vi "rad_Retrieve Application Image From Target.vi"(5 "password":string, 7 "App Images Temp Folder":path=path "C:/dev/Architectures/Reference Designs/Application Deployment and Replication/Application Deployment Utility/trunk/source/Application Images/_temp", 8 "error in (no error)":errorcluster, 10 "Target settings":T1={"Hostname"="", "Serial number"="", "Product name"="", "Product code"=0, "System status"="", "Credential type"=enum."None/Unlocked", "User added?"=FALSE, "Primary NIC"={"MAC address"="", "IP Address Request Mode"=2, "IP address"="", "Subnet mask"="", "Gateway"="", "DNS server"=""}} {"Primary NIC"."IP Address Request Mode" items=["Static"=1, "DHCP/Link-Local"=2, "Link-Local Only"=4, "DHCP Only"=8]}, 11 "App Images Folder":path) -> (0 "error out":errorcluster, 2 "Cancelled":bool, 3 "New App Image Path":path)   [LabVIEW 2020]
uses:
  TypeDefs/rad_Retrieve Application Image States.ctl
  TypeDefs/rad_FPGA Flash Properties.ctl
  TypeDefs/rad_FPGA Properties.ctl
  TypeDefs/rad_Application Image Properties.ctl
  TypeDefs/rad_Deployment Status Data Type.ctl
  TypeDefs/rad_Deployment Progress Data Type.ctl
  TypeDefs/rad_Deployment Notifiers.ctl
  TypeDefs/rad_App Images Settings.ctl
  Targets/TypeDefs/rad_Target Information.ctl
  Targets/TypeDefs/rad_Target Network Settings.ctl
panel:
  in  "State Data":T6
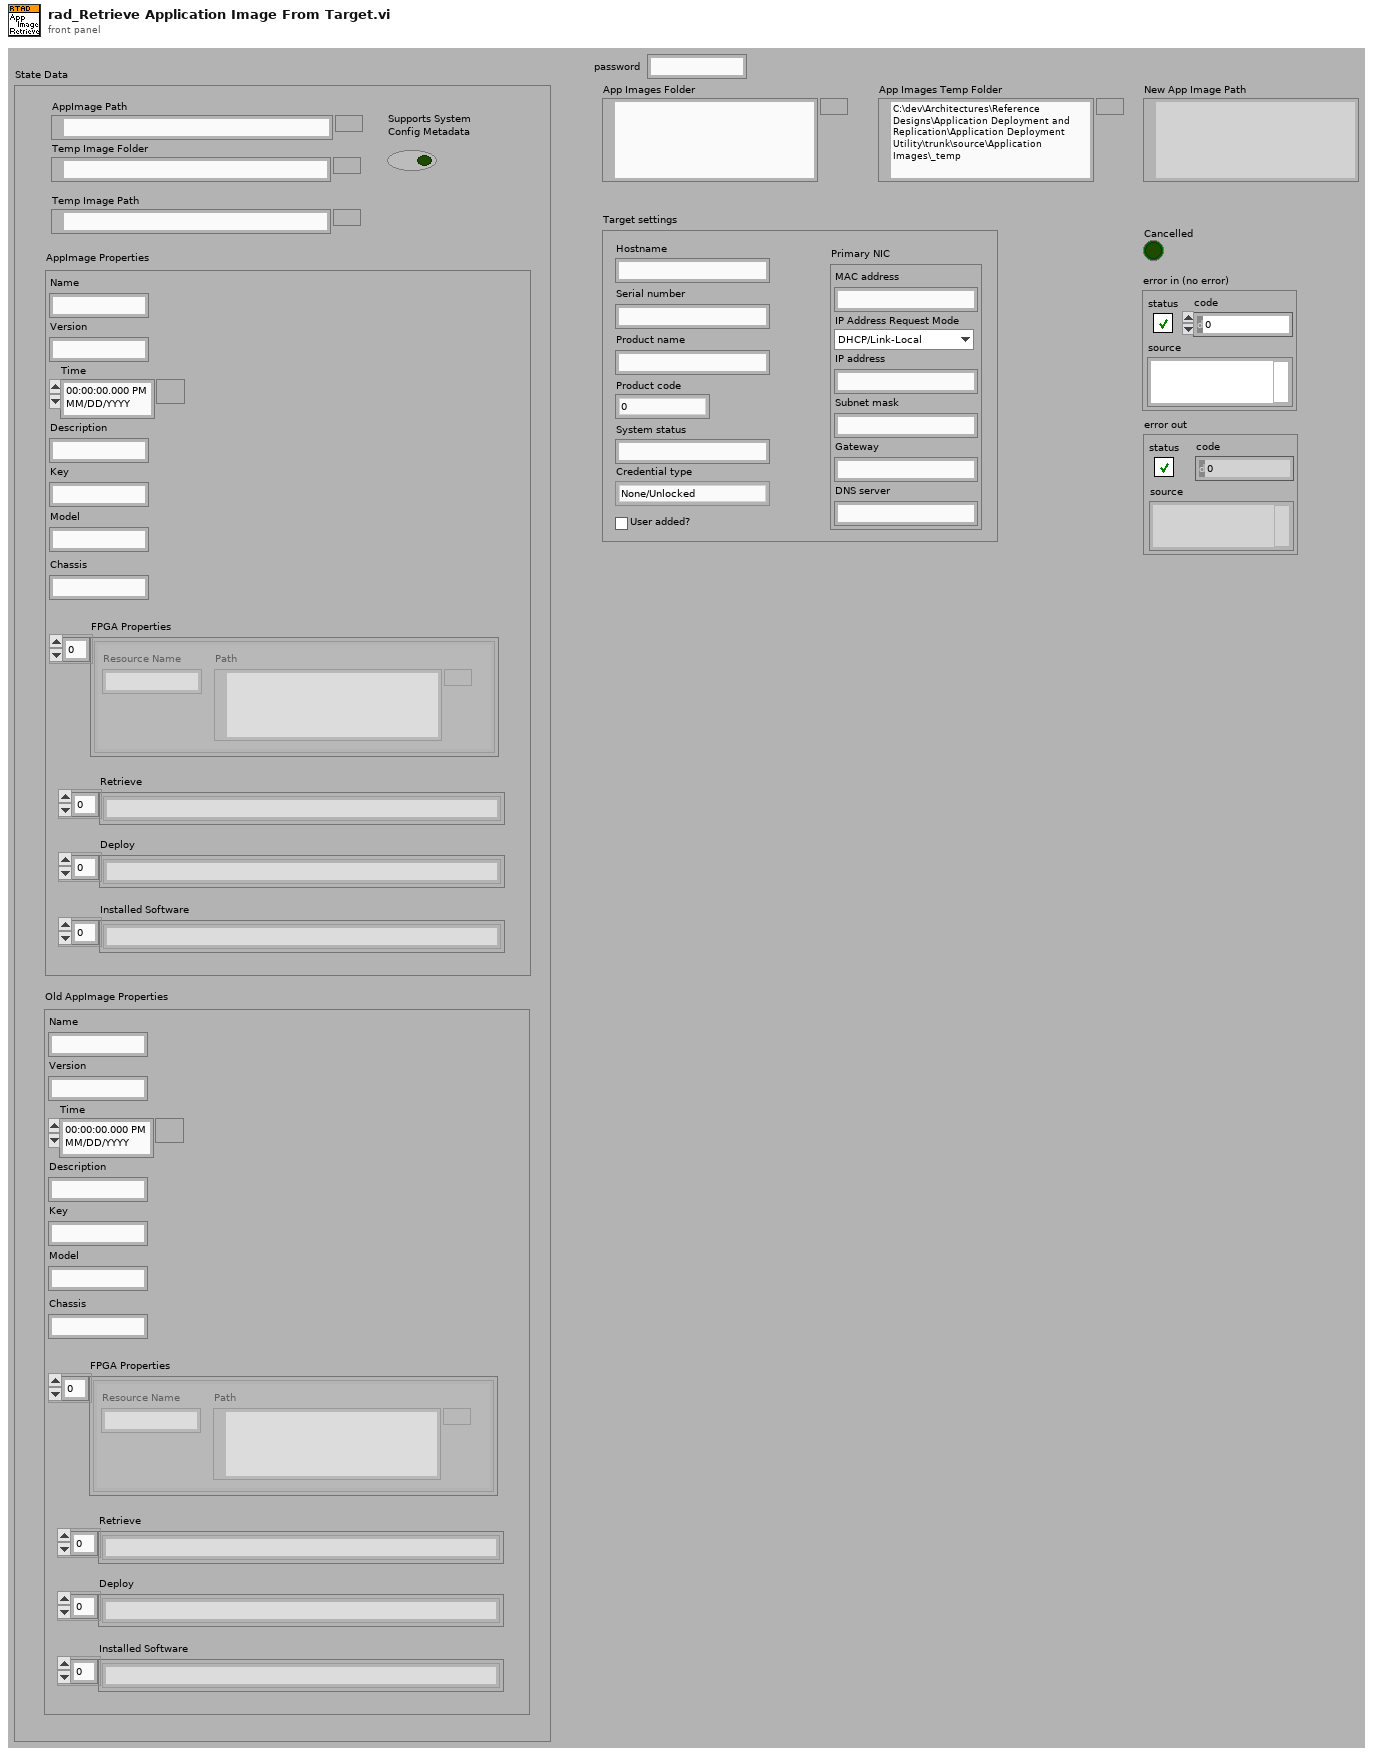
[diagram p1: front panel]
types:
  T1 = typedef "rad_Target Information.ctl" = cluster{"Hostname":string, "Serial number":string, "Product name":string, "Product code":i32, "System status":string, "Credential type":enum16{"None/Unlocked", "FTP Password", "NIAuth Credentials"}, "User added?":bool, "Primary NIC":T2}
  T2 = typedef "rad_Target Network Settings.ctl" = cluster{"MAC address":string, "IP Address Request Mode":i32, "IP address":string, "Subnet mask":string, "Gateway":string, "DNS server":string}
  T3 = typedef "rad_Application Image Properties.ctl" = cluster{"Name":string, "Version":string, "Time":timestamp, "Description":string, "Key":string, "Chassis":string, "FPGA Properties":T4, "Model":string, "Retrieve":string[], "Deploy":string[], "Installed Software":string[]}
  T4 = typedef "rad_FPGA Properties.ctl" = T5[]
  T5 = typedef "rad_FPGA Flash Properties.ctl" = cluster{"Resource Name":string, "Path":path}
  T6 = cluster{"AppImage Path":path, "Temp Image Folder":path, "AppImage Properties":T3, "App Image Info File Path":path, "New Image?":bool, "Selected Existing Image":path, "Bitfiles Modified?":bool, "Old AppImage Properties":T3, "Temp Image Path":path, "Supports System\nConfig Metadata":bool}
  T7 = typedef "rad_Retrieve Application Image States.ctl" = enum16{"Verify App Image Directory", "Get Target's Image Info", "Select Image Prop. Source", "Find Existing Disk Image", "Get Disk Image Properties", "Create New Image", "Set Image Properties", "Get Image Save Location", "GetInstalledSoftware", "Create App Image Info File", "Deploy New Files to Target", "Retrieve Application Image", "PackageImage", "Cleanup", "Exit"}
  T8 = typedef "rad_App Images Settings.ctl" = cluster{"App Images Folder":path, "App Images Temp Folder":path, "CurrentVersion":string}
  T9 = enum16{"None/Unlocked", "FTP Password", "NIAuth Credentials"}
  T10 = typedef "rad_Deployment Notifiers.ctl" = cluster{"Status":refnum<notifier>, "Progress":refnum<notifier>}
  T11 = typedef "rad_Deployment Progress Data Type.ctl" = i8
  T12 = typedef "rad_Deployment Status Data Type.ctl" = string
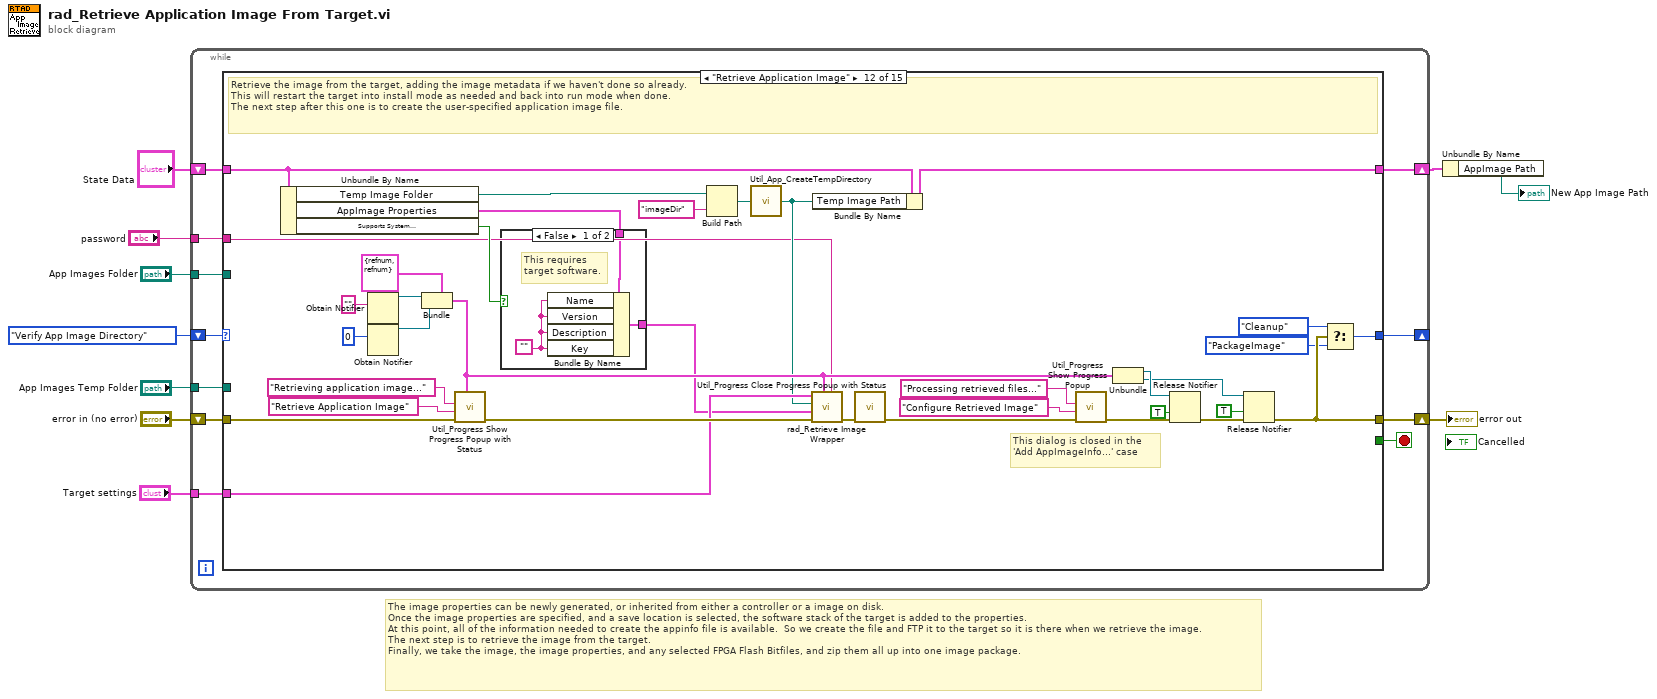
[diagram p0: block diagram]
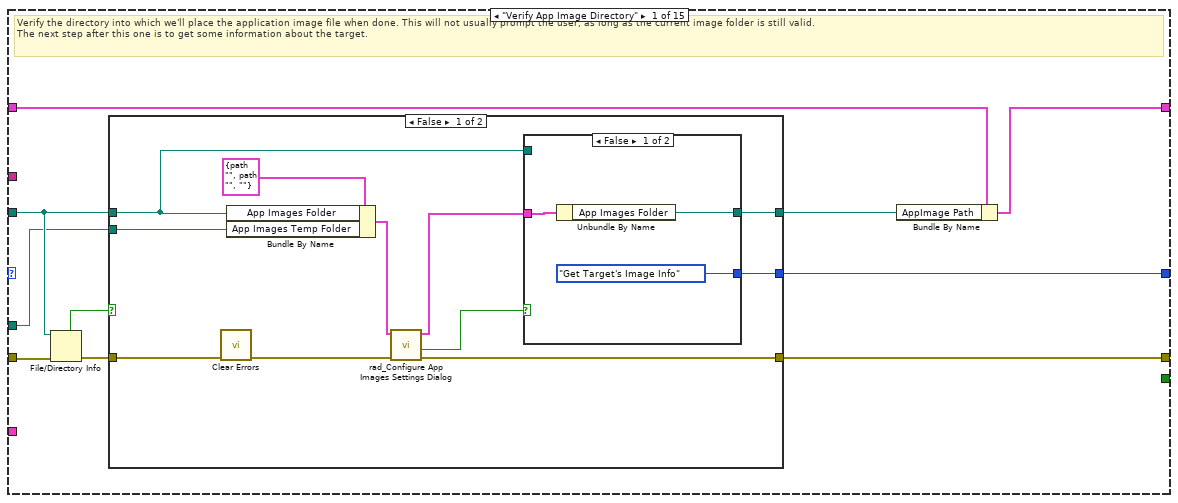
[diagram p2: hidden frame]
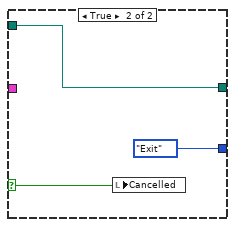
[diagram p3: hidden frame]
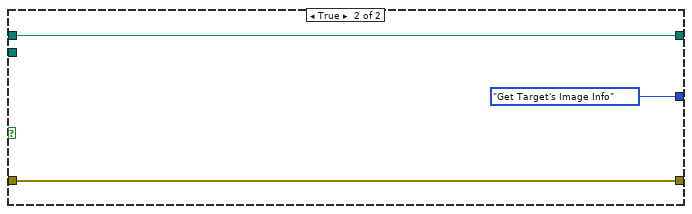
[diagram p4: hidden frame]
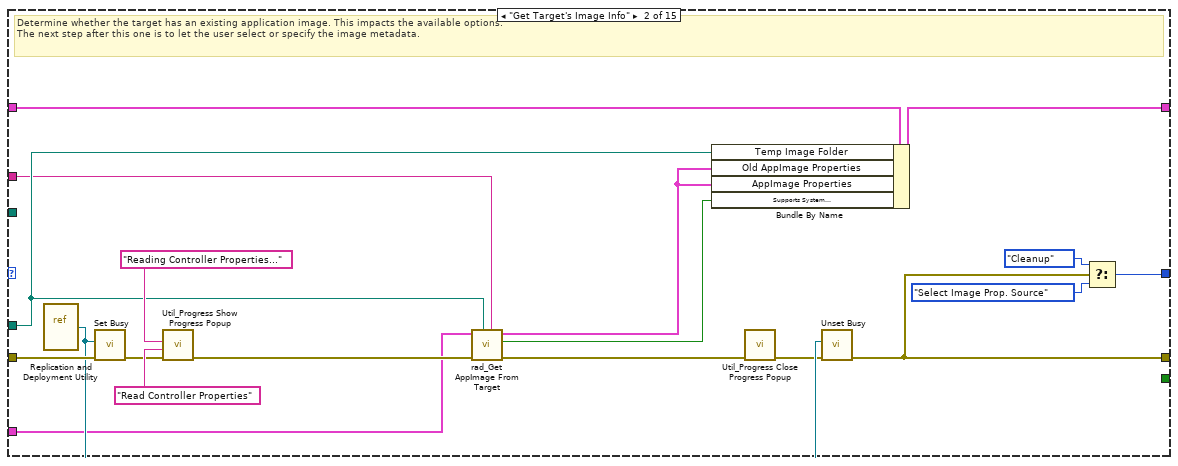
[diagram p5: hidden frame]
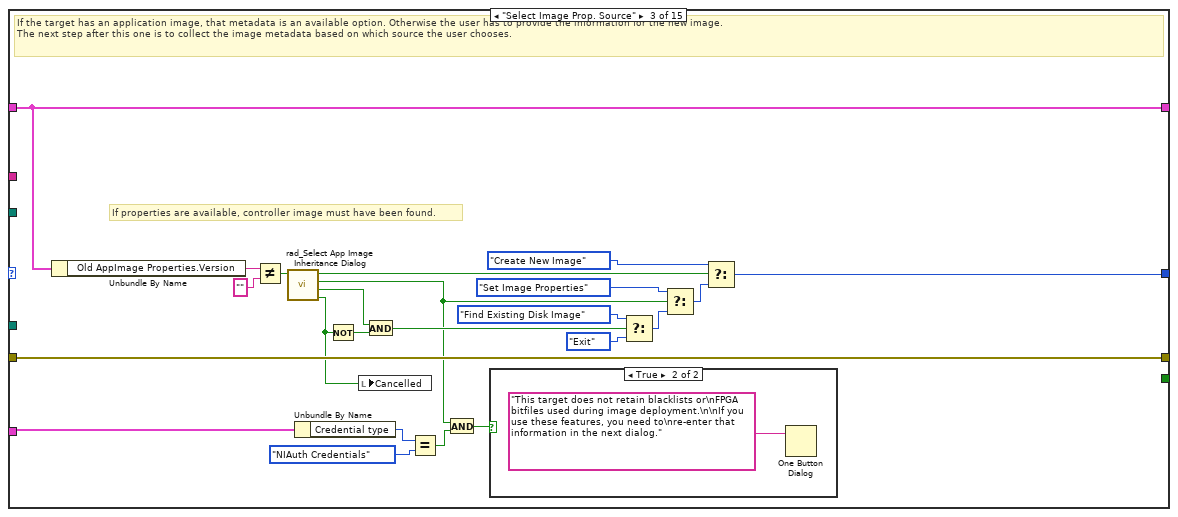
[diagram p6: hidden frame]
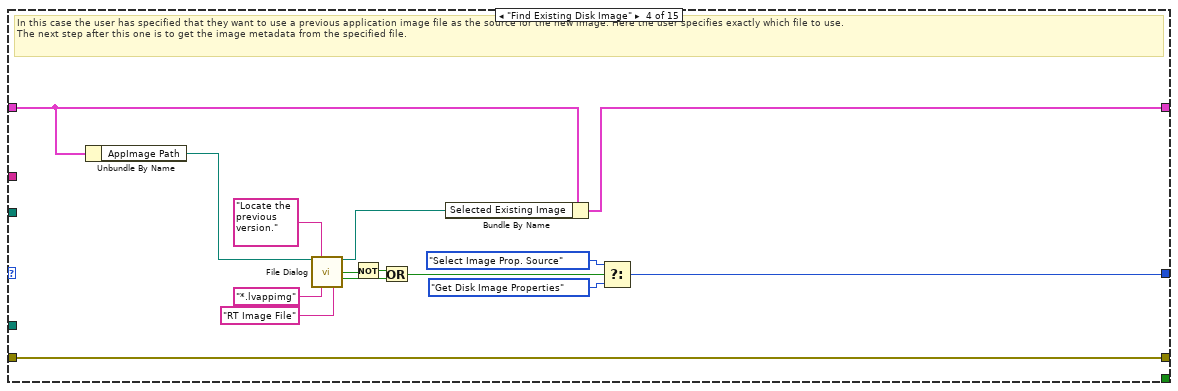
[diagram p8: hidden frame]
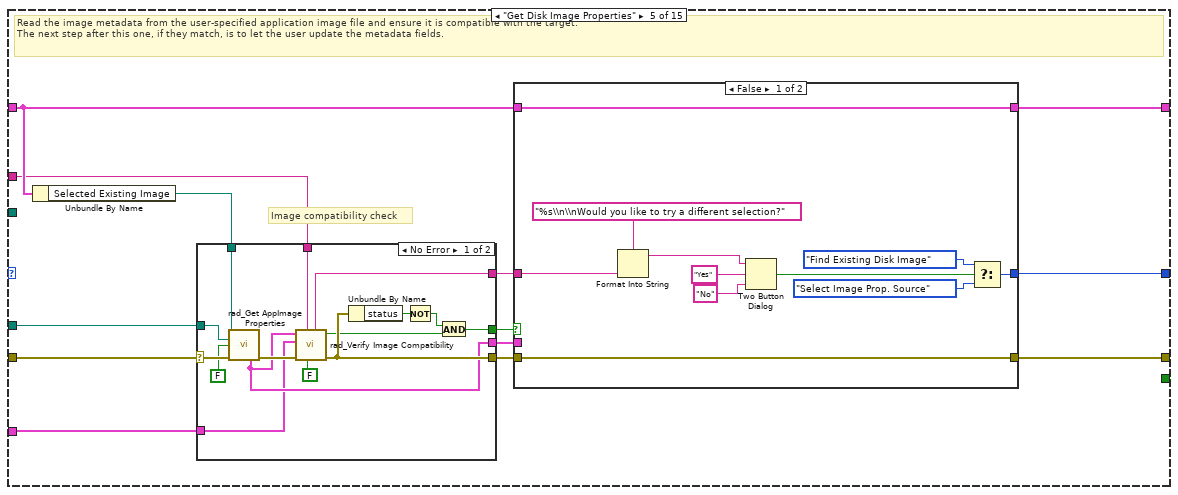
[diagram p9: hidden frame]
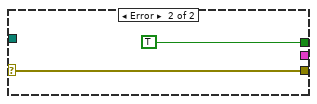
[diagram p10: hidden frame]
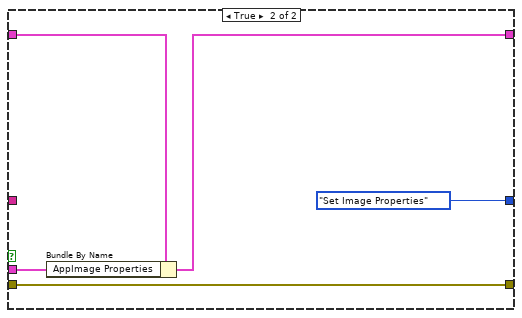
[diagram p11: hidden frame]
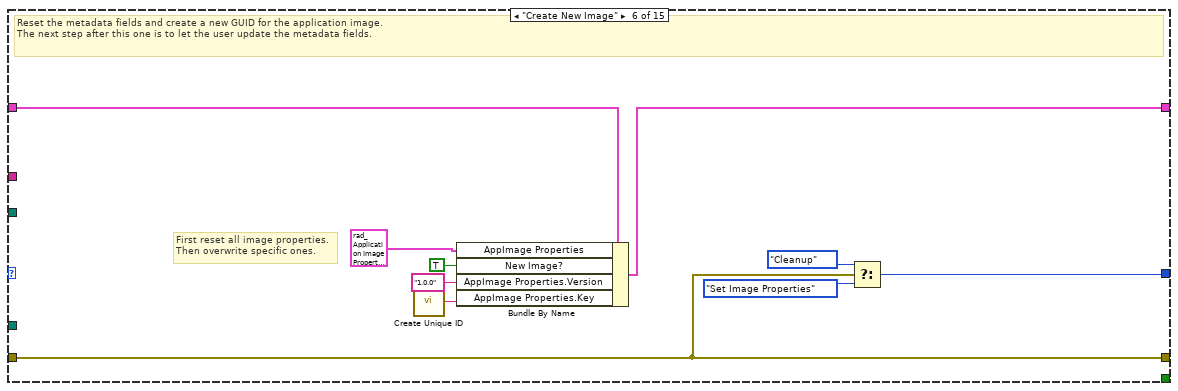
[diagram p12: hidden frame]
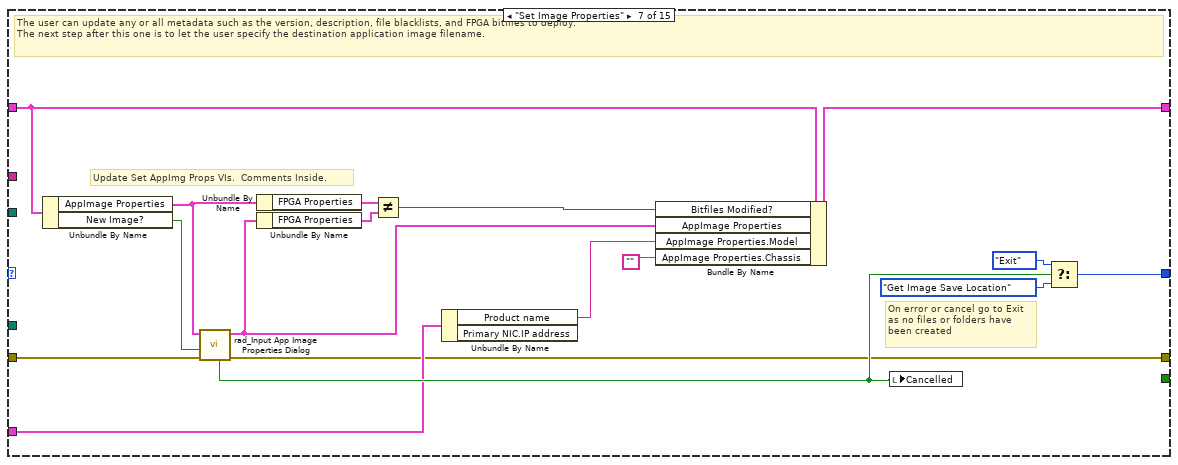
[diagram p13: hidden frame]
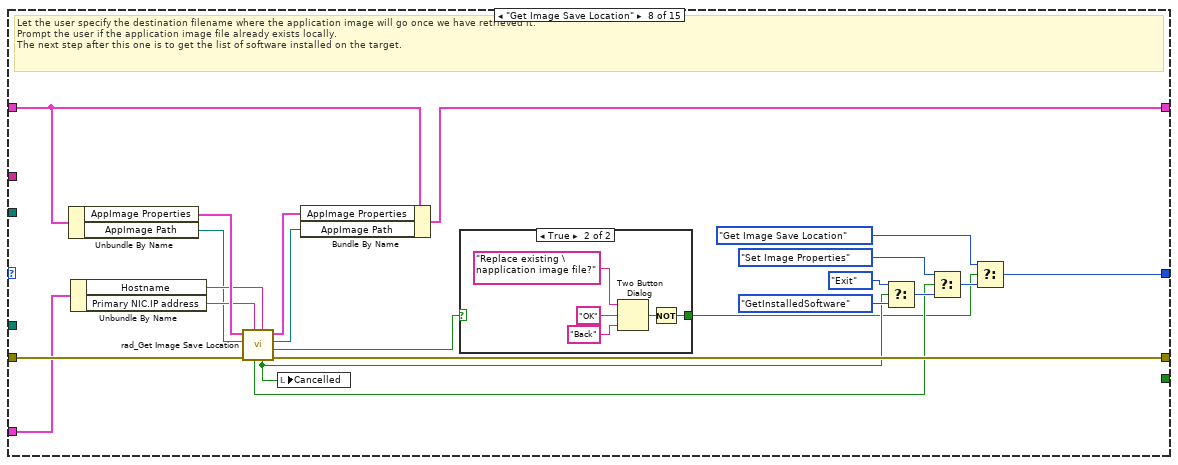
[diagram p14: hidden frame]
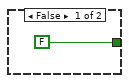
[diagram p15: hidden frame]
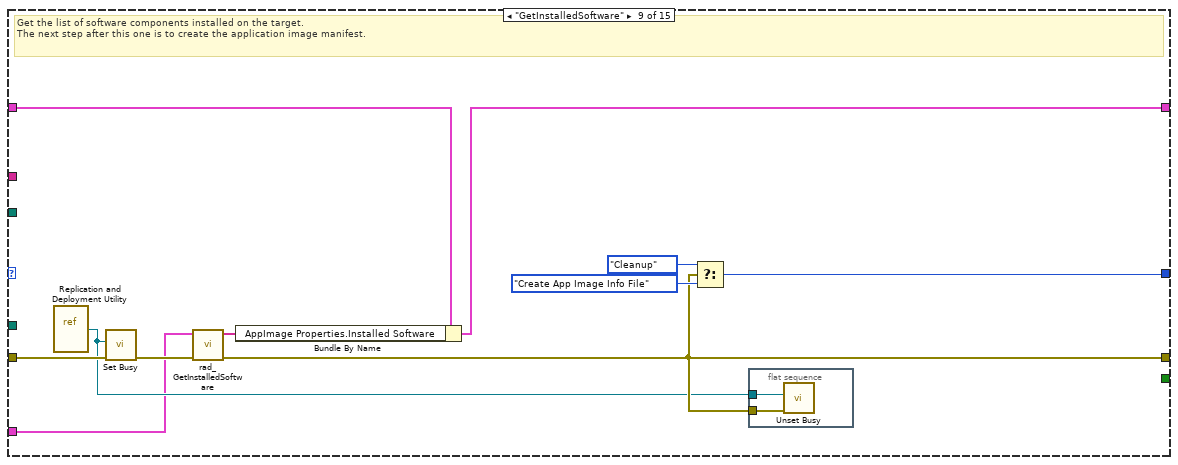
[diagram p16: hidden frame]
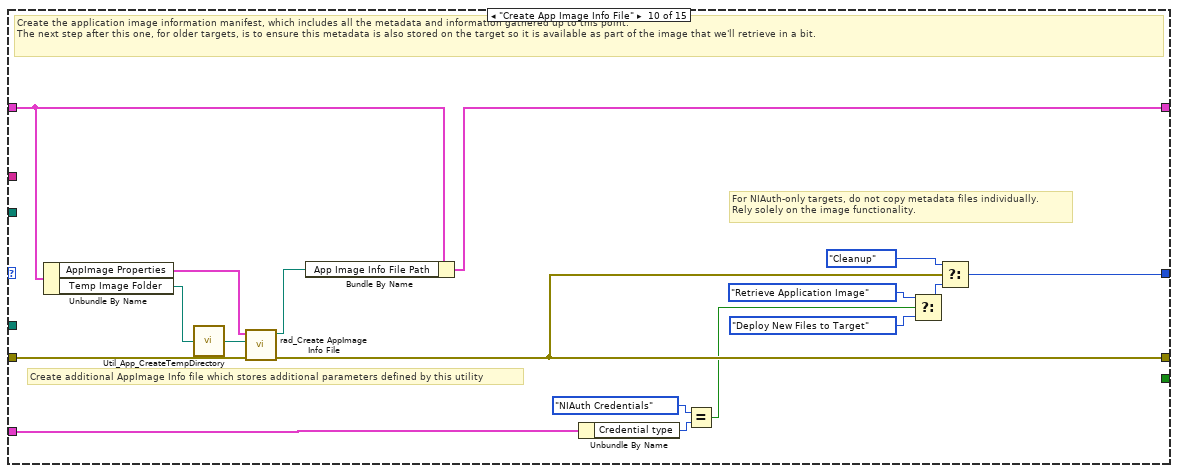
[diagram p17: hidden frame]
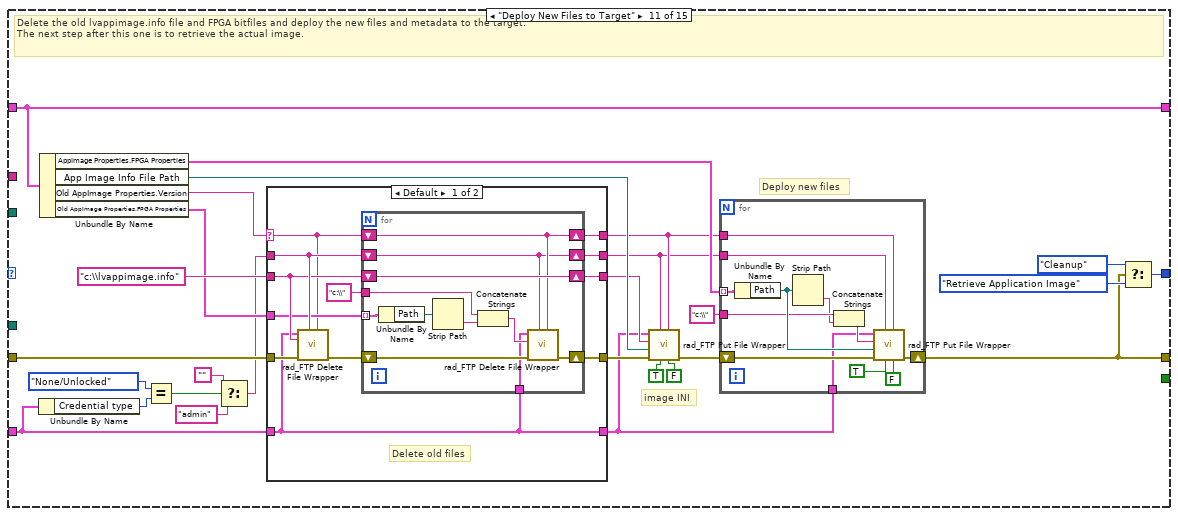
[diagram p18: hidden frame]
diagram:
  # "The image properties can be newly generated, or inherited from either a controller or a image on disk.\nOnce the image properties are specified, and a save location is selected, the software stack of the target is added to the properties.\nAt this point, all of the information needed to create the appinfo file is available.  So we create the file and FTP it to the target so it is there when we retrieve the image.\nThe next step is to retrieve the image from the target.\nFinally, we take the image, the image properties, and any selected FPGA Flash Bitfiles, and zip them all up into one image package."
  n1 = while {
    shift-right: [w20] -> _
    shift-left: rad_Retrieve_Application_Image_States."Verify App Image Directory" ("Retrieve App Images States") -> [w21]
    shift-right: [w17] -> w6
    shift-left: "State Data" -> [w18]
    shift-right: [w15] -> w7
    shift-left: "error in (no error)" -> [w16]
    tunnel: "App Images Folder" -> [w14]
    tunnel: "App Images Temp Folder" -> [w13]
    tunnel: "Target settings" -> [w12]
    tunnel: "password" -> [w11]
    stop <- w19 stop-if-true
    n2 = case shown="\"Retrieve Application Image\"" w21 {
      tunnel: [w25 w69 w81 w108 w121 w162 w182 w188 w217 w240 w252 w341 rad_Retrieve_Application_Image_States."Cleanup" ("Retrieve App Images States") rad_Retrieve_Application_Image_States."Exit" ("Retrieve App Images States") _] -> w20
      tunnel: [_ _ _ _ _ _ _ _ _ _ _ _ _ _ TRUE] -> w19
      tunnel: w18 -> [w24 w64 w93 w96 w118 w158 w177 w202 w220 w235 w267 w339 w351 w361 w375]
      tunnel: [w23 w68 w93 w107 w114 w165 w178 w201 w219 w237 w267 w340 w351 w361 w375] -> w17
      tunnel: w16 -> [w31 w63 w82 w109 w120 w156 w181 w204 w214 w233 w257 w334 w353 w355 w378]
      tunnel: [w28 w61 w82 w109 w116 w156 w167 w197 w215 w238 w251 w322 w352 w357 w378] -> w15
      tunnel: w14 -> [w27 _ _ _ _ _ _ _ _ _ _ _ _ _ _]
      tunnel: w13 -> [w26 w54 _ _ w115 _ _ _ _ _ _ _ _ _ _]
      tunnel: w12 -> [_ w55 w76 _ w111 _ w168 w186 w211 w227 w248 w315 _ _ _]
      tunnel: w11 -> [_ w52 _ _ w110 _ _ _ _ _ _ w308 _ _ _]
      frame "Verify App Image Directory" {
        # "Verify the directory into which we'll place the application image file when done. This will not usually prompt the user, as long as the current image folder is still valid.\nThe next step after this one is to get some information about the target."
        n3 = File/Directory Info(path=w27, error in=w31) -> (directory=w30:bool, error out=w29:errorcluster)  [unwired: 5 out]
        n4 = case shown="False" w30 {
          tunnel: w29 -> [w42 w51]
          tunnel: [w40 w51] -> w28
          tunnel: w27 -> [w32 w49]
          tunnel: w26 -> [w41 _]
          tunnel: [w37 rad_Retrieve_Application_Image_States."Get Target's Image Info" ("Retrieve App Images States")] -> w25
          tunnel: [w33 w49] -> w22
          frame False {
            n5 = call <vilib>:"Clear Errors.vi"("error in (no error)"=w42) -> ("error out"=w34:errorcluster)  [unwired: 5 in, 1 out]
            n6 = Bundle By Name(cluster=T8 {"App Images Folder"=path "", "App Images Temp Folder"=path "", "CurrentVersion"=""} ("App Images Settings"), "App Images Folder"=w32, "App Images Temp Folder"=w41) -> (w35:T8)
            n7 = call "rad_Configure App Images Settings Dialog.vi"("error in (no error)"=w34, "App Images Settings"=w35) -> ("error out"=w40:errorcluster, "Cancelled"=w39:bool, "App Images Settings"=w38:T8)  [unwired: 7 out]
            n8 = case shown="False" w39 {
              selector: w39 -> [_ w46]
              tunnel: w38 -> [w44 _]
              tunnel: [rad_Retrieve_Application_Image_States."Get Target's Image Info" ("Retrieve App Images States") rad_Retrieve_Application_Image_States."Exit" ("Retrieve App Images States")] -> w37
              tunnel: [w43 w47] -> w33
              tunnel: w32 -> [_ w47]
              frame False {
                n9 = Unbundle By Name(w44) -> ("App Images Folder"=w43:path)
              }
              frame True {
                n10 = local write "Cancelled"(w46) -> ()
              }
            }
          }
          frame True {
          }
        }
        n11 = Bundle By Name(cluster=w24, "AppImage Path"=w22) -> (w23:T6)
      }
      frame "Get Target's Image Info" {
        # "Determine whether the target has an existing application image. This impacts the available options.\nThe next step after this one is to let the user select or specify the image metadata."
        n12 = vi-ref "Replication and Deployment Utility.vi"() -> (w60:refnum<vi>)
        n13 = call <vilib>:"Set Busy.vi"("error in (no error)"=w63, "VI reference (current VI)"=w60) -> ("error out"=w62:errorcluster)  [unwired: 8 in, 1 out]
        n14 = call "Util_Progress Show Progress Popup.vi"("error in (no error)"=w62, "Title"="Read Controller Properties", "Message"="Reading Controller Properties...") -> ("error out"=w58:errorcluster)  [unwired: 8 in]
        n15 = call "rad_Get AppImage From Target.vi"("password"=w52, "Temp Folder"=w54, "error in (no error)"=w58, "Target settings"=w55) -> ("error out"=w57:errorcluster, "Supports System\nConfig Metadata"=w53:bool, "AppImage Properties"=w56:T3)  [unwired: 5 in]
        n16 = Bundle By Name(cluster=w64, "Temp Image Folder"=w54, "Old AppImage Properties"=w56, "AppImage Properties"=w56, "Supports System\nConfig Metadata"=w53) -> (w68:T6)
        n17 = call "Util_Progress Close Progress Popup.vi"("error in (no error)"=w57) -> ("error out"=w59:errorcluster)  [unwired: 10 in]
        n18 = call <vilib>:"Unset Busy.vi"("error in (no error)"=w59, "VI reference (current VI)"=w60) -> ("error out"=w61:errorcluster)  [unwired: 9 in]
        n19 = Select(t=rad_Retrieve_Application_Image_States."Cleanup", s=w61, f=rad_Retrieve_Application_Image_States."Select Image Prop. Source" ("Retrieve App Images States")) -> (s? t:f=w69:T7)
      }
      frame "Select Image Prop. Source" {
        # "If properties are available, controller image must have been found."
        # "If the target has an application image, that metadata is an available option. Otherwise the user has to provide the information for the new image.\nThe next step after this one is to collect the image metadata based on which source the user chooses."
        n20 = Unbundle By Name(w93) -> ("Old AppImage Properties.Version"=w92:string)
        n21 = Not Equal?(x=w92, y="") -> (x != y?=w90:bool)
        n22 = call "rad_Select App Image Inheritance Dialog.vi"("Controller Image Available?"=w90) -> ("Cancel"=w77:bool, "Disc Image"=w80:bool, "Controller Image"=w72:bool, "New Image"=w89:bool)  [unwired: 7 in]
        n23 = Unbundle By Name(w76) -> ("Credential type"=w75:T9)
        n24 = Not(x=w77) -> (.not. x?=w79:bool)
        n25 = local write "Cancelled"(w77) -> ()
        n26 = And(x=w80, y=w79) -> (x .and. y?=w78:bool)
        n27 = Equal?(x=w75, y=T9."NIAuth Credentials" ("Credential type")) -> (x = y?=w73:bool)
        n28 = And(x=w72, y=w73) -> (x .and. y?=w71:bool)
        n29 = case shown="True" w71 {
          frame False {
          }
          frame True {
            n30 = One Button Dialog(message="This target does not retain blacklists or\nFPGA bitfiles used during image deployment.\n\nIf you use these features, you need to\nre-enter that information in the next dialog.") -> ()  [unwired: 1 in, 1 out]
          }
        }
        n31 = Select(t=rad_Retrieve_Application_Image_States."Find Existing Disk Image" ("Retrieve App Images States"), s=w78, f=rad_Retrieve_Application_Image_States."Exit" ("Retrieve App Images States")) -> (s? t:f=w84:T7)
        n32 = Select(t=rad_Retrieve_Application_Image_States."Set Image Properties" ("Retrieve App Images States"), s=w72, f=w84) -> (s? t:f=w86:T7)
        n33 = Select(t=rad_Retrieve_Application_Image_States."Create New Image" ("Retrieve App Images States"), s=w89, f=w86) -> (s? t:f=w81:T7)
      }
      frame "Find Existing Disk Image" {
        # "In this case the user has specified that they want to use a previous application image file as the source for the new image. Here the user specifies exactly which file to use.\nThe next step after this one is to get the image metadata from the specified file."
        n34 = Unbundle By Name(w96) -> ("AppImage Path"=w95:path)
        n35 = call "File Dialog"("start path"=w95, "prompt"="Locate the previous version.", "pattern (all files)"="*.lvappimg", "pattern label"="RT Image File") -> ("selected path"=w97:path, "exists"=w104:bool, "cancelled"=w102:bool)  [unwired: 8 in, 1 out]
        n36 = Not(x=w104) -> (.not. x?=w103:bool)
        n37 = Or(x=w103, y=w102) -> (x .or. y?=w100:bool)
        n38 = Bundle By Name(cluster=w96, "Selected Existing Image"=w97) -> (w107:T6)
        n39 = Select(t=rad_Retrieve_Application_Image_States."Select Image Prop. Source" ("f"), s=w100, f=rad_Retrieve_Application_Image_States."Get Disk Image Properties") -> (s? t:f=w108:T7)
      }
      frame "Get Disk Image Properties" {
        # "Image compatibility check"
        # "Read the image metadata from the user-specified application image file and ensure it is compatible with the target.\nThe next step after this one, if they match, is to let the user update the metadata fields."
        n40 = Unbundle By Name(w118) -> ("Selected Existing Image"=w122:path)
        n41 = case shown="No Error" w120 {
          selector: w120 -> [w129 w139]
          tunnel: w115 -> [w130 _]
          tunnel: w122 -> [w131 _]
          tunnel: [w137 w139] -> w117
          tunnel: [w135 TRUE] -> w119
          tunnel: [w126 _] -> w113
          tunnel: w111 -> [w125 _]
          tunnel: [w124 _] -> w112
          tunnel: w110 -> [w123 _]
          frame No Error {
            n42 = call "rad_Get AppImage Properties.vi"("AppImage Path"=w131, "App Image Temp Folder"=w130, "Show FP"=FALSE, "error in (no error)"=w129) -> ("AppImage Properties"=w126:T3, "error out"=w128:errorcluster)  [unwired: 5 in, 5 out]
            n43 = call "rad_Verify Image Compatibility.vi"("Require Identical Chassis?"=FALSE, "Password"=w123, "error in (no error)"=w128, "Target address"=w125, "AppImage Properties"=w126) -> ("error out"=w137:errorcluster, "Compatible?"=w134:bool, "Status message"=w124:string)  [unwired: 4 in]
            n44 = Unbundle By Name(w137) -> ("status"=w136:bool)
            n45 = Not(x=w136) -> (.not. x?=w133:bool)
            n46 = And(x=w133, y=w134) -> (x .and. y?=w135:bool)
          }
          frame Error {
          }
        }
        n47 = case shown="False" w119 {
          tunnel: [w145 rad_Retrieve_Application_Image_States."Set Image Properties" ("Retrieve App Images States")] -> w121
          tunnel: w118 -> [w143 w155]
          tunnel: w117 -> [w144 w151]
          tunnel: [w144 w151] -> w116
          tunnel: [w143 w153] -> w114
          tunnel: w113 -> [_ w152]
          tunnel: w112 -> [w141 _]
          frame False {
            n48 = Format Into String(format string="%s\\n\\nWould you like to try a different selection?" ("message"), w141) -> (resulting string=w140:string)  [unwired: 2 in, 1 out]
            n49 = Two Button Dialog(message=w140, 1:"No" ("F button name (\"Cancel\")"), 2:"Yes" ("T button name (\"OK\")")) -> (T button?=w147:bool)
            n50 = Select(t=rad_Retrieve_Application_Image_States."Find Existing Disk Image" ("Retrieve App Images States"), s=w147, f=rad_Retrieve_Application_Image_States."Select Image Prop. Source" ("Retrieve App Images States")) -> (s? t:f=w145:T7)
          }
          frame True {
            n51 = Bundle By Name(cluster=w155, "AppImage Properties"=w152) -> (w153:T6)
          }
        }
      }
      frame "Create New Image" {
        # "First reset all image properties.\nThen overwrite specific ones."
        # "Reset the metadata fields and create a new GUID for the application image.\nThe next step after this one is to let the user update the metadata fields."
        n52 = call "Create Unique ID.vi"() -> ("ID String"=w161:string)  [unwired: 1 in]
        n53 = Bundle By Name(cluster=w158, "AppImage Properties"=T3 {"Name"="", "Version"="", "Time"=timestamp(0 s since 1904-01-01), "Description"="", "Key"="", "Chassis"="", "FPGA Properties"=[], "Model"="", "Retrieve"=[], "Deploy"=[], "Installed Software"=[]}, "New Image?"=TRUE, "AppImage Properties.Version"="1.0.0", "AppImage Properties.Key"=w161) -> (w165:T6)
        n54 = Select(t=rad_Retrieve_Application_Image_States."Cleanup", s=w156, f=rad_Retrieve_Application_Image_States."Set Image Properties" ("Retrieve App Images States")) -> (s? t:f=w162:T7)
      }
      frame "Set Image Properties" {
        # "Update Set AppImg Props VIs.  Comments Inside."
        # "On error or cancel go to Exit\nas no files or folders have\nbeen created"
        # "The user can update any or all metadata such as the version, description, file blacklists, and FPGA bitfiles to deploy.\nThe next step after this one is to let the user specify the destination application image filename."
        n55 = Unbundle By Name(w177) -> ("AppImage Properties"=w172:T3, "New Image?"=w173:bool)
        n56 = call "rad_Input App Image Properties Dialog.vi"("error in (no error)"=w181, "New Image?"=w173, "AppImage Properties"=w172) -> ("error out"=w167:errorcluster, "AppImage Properties"=w170:T3, "Cancelled"=w171:bool)  [unwired: 4 in, 2 out]
        n57 = Unbundle By Name(w172) -> ("FPGA Properties"=w176:T4)
        n58 = Unbundle By Name(w170) -> ("FPGA Properties"=w175:T4)
        n59 = Not Equal?(x=w176, y=w175) -> (x != y?=w174:bool)
        n60 = Unbundle By Name(w168) -> ("Product name"=w169:string)  [unwired: 1 out]
        n61 = Bundle By Name(cluster=w177, "Bitfiles Modified?"=w174, "AppImage Properties"=w170, "AppImage Properties.Model"=w169, "AppImage Properties.Chassis"="") -> (w178:T6)
        n62 = local write "Cancelled"(w171) -> ()
        n63 = Select(t=rad_Retrieve_Application_Image_States."Exit" ("Retrieve App Images States"), s=w171, f=rad_Retrieve_Application_Image_States."Get Image Save Location" ("Retrieve App Images States")) -> (s? t:f=w182:T7)
      }
      frame "Get Image Save Location" {
        # "Let the user specify the destination filename where the application image will go once we have retrieved it.\nPrompt the user if the application image file already exists locally.\nThe next step after this one is to get the list of software installed on the target."
        n64 = Unbundle By Name(w202) -> ("AppImage Properties"=w203:T3, "AppImage Path"=w183:path)
        n65 = Unbundle By Name(w186) -> ("Hostname"=w185:string, "Primary NIC.IP address"=w184:string)
        n66 = call "rad_Get Image Save Location.vi"("Host Name"=w185, "IP Address"=w184, "error in (no error)"=w204, "Starting Path"=w183, "AppImage Properties"=w203) -> ("error out"=w197:errorcluster, "exists"=w198:bool, "Application Image Path"=w192:path, "AppImage Properties"=w200:T3, "Cancelled"=w191:bool, "Back"=w194:bool)  [unwired: 1 in]
        n67 = local write "Cancelled"(w191) -> ()
        n68 = Bundle By Name(cluster=w202, "AppImage Properties"=w200, "AppImage Path"=w192) -> (w201:T6)
        n69 = case shown="True" w198 {
          tunnel: [FALSE ("T button?") w206] -> w189
          frame False {
          }
          frame True {
            n70 = Two Button Dialog(message="Replace existing \napplication image file?", 1:"Back" ("F button name (\"Cancel\")"), 2:"OK" ("T button name (\"OK\")")) -> (T button?=w209:bool)
            n71 = Not(x=w209) -> (.not. x?=w206:bool)
          }
        }
        n72 = Select(t=rad_Retrieve_Application_Image_States."Exit" ("Retrieve App Images States"), s=w191, f=rad_Retrieve_Application_Image_States."GetInstalledSoftware" ("Retrieve App Images States")) -> (s? t:f=w195:T7)
        n73 = Select(t=rad_Retrieve_Application_Image_States."Set Image Properties", s=w194, f=w195) -> (s? t:f=w190:T7)
        n74 = Select(t=rad_Retrieve_Application_Image_States."Get Image Save Location", s=w189, f=w190) -> (s? t:f=w188:T7)
      }
      frame "GetInstalledSoftware" {
        # "Get the list of software components installed on the target.\nThe next step after this one is to create the application image manifest."
        n75 = vi-ref "Replication and Deployment Utility.vi"() -> (w212:refnum<vi>)
        n76 = call <vilib>:"Set Busy.vi"("error in (no error)"=w214, "VI reference (current VI)"=w212) -> ("error out"=w213:errorcluster)  [unwired: 8 in, 1 out]
        n77 = call "rad_GetInstalledSoftware.vi"("error in (no error)"=w213, "Target settings"=w211) -> ("error out"=w215:errorcluster, "installedSoftware"=w221:string[])  [unwired: 8 in]
        n78 = Bundle By Name(cluster=w220, "AppImage Properties.Installed Software"=w221) -> (w219:T6)
        n79 = Select(t=rad_Retrieve_Application_Image_States."Cleanup", s=w215, f=rad_Retrieve_Application_Image_States."Create App Image Info File" ("Retrieve App Images States")) -> (s? t:f=w217:T7)
        n80 = flat-sequence {
          tunnel: w215 -> [w223]
          tunnel: w212 -> [w222]
          frame #0 {
            n81 = call <vilib>:"Unset Busy.vi"("error in (no error)"=w223, "VI reference (current VI)"=w222) -> ()  [unwired: 9 in, 1 out]
          }
        }
      }
      frame "Create App Image Info File" {
        # "For NIAuth-only targets, do not copy metadata files individually.\nRely solely on the image functionality."
        # "Create additional AppImage Info file which stores additional parameters defined by this utility"
        # "Create the application image information manifest, which includes all the metadata and information gathered up to this point.\nThe next step after this one, for older targets, is to ensure this metadata is also stored on the target so it is available as part of the image that we'll retrieve in a bit."
        n82 = Unbundle By Name(w235) -> ("AppImage Properties"=w234:T3, "Temp Image Folder"=w224:path)
        n83 = call "Util_App_CreateTempDirectory.vi"("TempFolderPath"=w224) -> ("TempFolderPath_out"=w232:path)
        n84 = call "rad_Create AppImage Info File.vi"("error in (no error)"=w233, "Temp Image Folder"=w232, "AppImage Properties"=w234) -> ("error out"=w238:errorcluster, "App Image Info file path"=w236:path)  [unwired: 7 in]
        n85 = Bundle By Name(cluster=w235, "App Image Info File Path"=w236) -> (w237:T6)
        n86 = Unbundle By Name(w227) -> ("Credential type"=w229:T9)
        n87 = Equal?(x=T9."NIAuth Credentials" ("Credential type"), y=w229) -> (x = y?=w226:bool)
        n88 = Select(t=rad_Retrieve_Application_Image_States."Retrieve Application Image" ("Retrieve App Images States"), s=w226, f=rad_Retrieve_Application_Image_States."Deploy New Files to Target" ("Retrieve App Images States")) -> (s? t:f=w231:T7)
        n89 = Select(t=rad_Retrieve_Application_Image_States."Cleanup" ("Retrieve App Images States"), s=w238, f=w231) -> (s? t:f=w240:T7)
      }
      frame "Deploy New Files to Target" {
        # "Deploy new files"
        # "image INI"
        # "Delete the old lvappimage.info file and FPGA bitfiles and deploy the new files and metadata to the target.\nThe next step after this one is to retrieve the actual image."
        n90 = Unbundle By Name(w248) -> ("Credential type"=w246:T9)
        n91 = Unbundle By Name(w267) -> ("AppImage Properties.FPGA Properties"=w263:T4, "App Image Info File Path"=w266:path, "Old AppImage Properties.Version"=w241:string, "Old AppImage Properties.FPGA Properties"=w250:T4)
        n92 = Equal?(x=T9."None/Unlocked" ("Credential type"), y=w246) -> (x = y?=w244:bool)
        n93 = Select(t="", s=w244, f="admin" ("user")) -> (s? t:f=w249:string)
        n94 = case shown="Default" w241 {
          selector: w241 -> [w268 w291]
          tunnel: [w278 w291] -> w261
          tunnel: w249 -> [w277 w295]
          tunnel: [w276 w295] -> w260
          tunnel: "c:\\lvappimage.info" ("remote path") -> [w274 w294]
          tunnel: [w275 w294] -> w258
          tunnel: w257 -> [w279 w293]
          tunnel: [w270 w293] -> w256
          tunnel: w250 -> [w272 _]
          tunnel: w248 -> [w269 w292]
          tunnel: [w269 w292] -> w247
          frame Default {
            # "Delete old files"
            n95 = call "rad_FTP Delete File Wrapper.vi"("password"=w268, "user (admin)"=w277, "error in (no error)"=w279, "remote path"=w274, "Target settings"=w269) -> ("error out"=w271:errorcluster)  [unwired: 6 in]
            n96 = for {
              shift-right: [w285] -> w270
              shift-left: w271 -> [w284]
              tunnel: w272 -> [w290] mode=indexing
              tunnel: "c:\\" ("remote path") -> [w288]
              shift-right: [w282] -> w278
              shift-left: w268 -> [w282]
              shift-right: [w281] -> w276
              shift-left: w277 -> [w281]
              shift-right: [w286] -> w275
              shift-left: w274 -> [w286]
              tunnel: w269 -> [w280]
              n97 = Unbundle By Name(w290) -> ("Path"=w289:path)
              n98 = Strip Path(path=w289) -> (name=w287:string)  [unwired: 1 out]
              n99 = Concatenate Strings(w288, w287) -> (w283:string)
              n100 = call "rad_FTP Delete File Wrapper.vi"("password"=w282, "user (admin)"=w281, "error in (no error)"=w284, "remote path"=w283, "Target settings"=w280) -> ("error out"=w285:errorcluster)  [unwired: 6 in]
            }
          }
          frame "" {
          }
        }
        n101 = call "rad_FTP Put File Wrapper.vi"("active (F)"=FALSE ("active (T)"), "password"=w261, "binary (T)"=TRUE ("binary (F)"), "user (admin)"=w260, "error in (no error)"=w256, "local path"=w266, "remote path"=w258, "Target settings"=w247) -> ("error out"=w264:errorcluster)  [unwired: 3 in]
        n102 = for {
          shift-right: [w306] -> w251
          shift-left: w264 -> [w307]
          tunnel: w261 -> [w305]
          tunnel: w260 -> [w304]
          tunnel: w263 -> [w303] mode=indexing
          tunnel: "c:\\" ("remote path") -> [w301]
          tunnel: w247 -> [w296]
          n103 = Unbundle By Name(w303) -> ("Path"=w302:path)
          n104 = Strip Path(path=w302) -> (name=w300:string)  [unwired: 1 out]
          n105 = Concatenate Strings(w301, w300) -> (w299:string)
          n106 = call "rad_FTP Put File Wrapper.vi"("active (F)"=FALSE ("active (T)"), "password"=w305, "binary (T)"=TRUE ("binary (F)"), "user (admin)"=w304, "error in (no error)"=w307, "local path"=w302, "remote path"=w299, "Target settings"=w296) -> ("error out"=w306:errorcluster)  [unwired: 3 in]
        }
        n107 = Select(t=rad_Retrieve_Application_Image_States."Cleanup" ("Retrieve App Images States"), s=w251, f=rad_Retrieve_Application_Image_States."Retrieve Application Image" ("Retrieve App Images States")) -> (s? t:f=w252:T7)
      }
      frame "Retrieve Application Image" {
        # "This dialog is closed in the 'Add AppImageInfo...' case"
        # "Retrieve the image from the target, adding the image metadata if we haven't done so already.\nThis will restart the target into install mode as needed and back into run mode when done.\nThe next step after this one is to create the user-specified application image file."
        n108 = Unbundle By Name(w339) -> ("Temp Image Folder"=w312:path, "AppImage Properties"=w310:T3, "Supports System\nConfig Metadata"=w311:bool)
        n109 = Obtain Notifier(notification data type=T12 "" ("status notifier data type")) -> (notifier out=w327:refnum<notifier>)  [unwired: 3 in, 2 out]
        n110 = Obtain Notifier(notification data type=T11 0 ("Progress")) -> (notifier out=w328:refnum<notifier>)  [unwired: 3 in, 2 out]
        n111 = Bundle(cluster=T10 {"Status"=refnum, "Progress"=refnum} ("Deployment Notifiers"), "Status"=w327, "Progress"=w328) -> (w326:T10)
        n112 = call "Util_Progress Show Progress Popup with Status.vi"("Deployment Notifiers"=w326, "error in (no error)"=w334, "Title"="Retrieve Application Image", "Message"="Retrieving application image...") -> ("error out"=w333:errorcluster)  [unwired: 7 in]
        n113 = case shown="False" w311 {
          tunnel: w310 -> [w345 w346]
          tunnel: [w343 w346] -> w309
          frame False {
            w344 = ""
            # "This requires\ntarget software."
            n114 = Bundle By Name(cluster=w345, "Name"=w344, "Version"=w344, "Description"=w344, "Key"=w344) -> (w343:T3)
          }
          frame True {
          }
        }
        n115 = Build Path(base path=w312, name or relative path="imageDir") -> (appended path=w318:path)
        n116 = call "Util_App_CreateTempDirectory.vi"("TempFolderPath"=w318) -> ("TempFolderPath_out"=w313:path)
        n117 = call "rad_Retrieve Image Wrapper.vi"("Password"=w308, "Deployment Notifiers"=w326, "error in (no error)"=w333, "AppImage Properties"=w309, "image file path"=w313, "Target settings"=w315) -> ("error out"=w317:errorcluster)  [unwired: 4 in, 1 out]
        n118 = Bundle By Name(cluster=w339, "Temp Image Path"=w313) -> (w340:T6)
        n119 = call "Util_Progress Close Progress Popup with Status.vi"("error in (no error)"=w317) -> ("error out"=w330:errorcluster)  [unwired: 10 in]
        n120 = call "Util_Progress Show Progress Popup.vi"("error in (no error)"=w330, "Title"="Configure Retrieved Image", "Message"="Processing retrieved files...") -> ("error out"=w316:errorcluster)  [unwired: 8 in]
        n121 = Unbundle(w326) -> ("Status"=w325:refnum<notifier>, "Progress"=w324:refnum<notifier>)
        n122 = Release Notifier(notifier=w325, force destroy? (F)=TRUE, error in (no error)=w316) -> (error out=w323:errorcluster)  [unwired: 2 out]
        n123 = Release Notifier(notifier=w324, force destroy? (F)=TRUE, error in (no error)=w323) -> (error out=w322:errorcluster)  [unwired: 2 out]
        n124 = Select(t=rad_Retrieve_Application_Image_States."Cleanup" ("Retrieve App Images States"), s=w322, f=rad_Retrieve_Application_Image_States."PackageImage" ("Retrieve App Images States")) -> (s? t:f=w341:T7)
      }
      frame "PackageImage" {
        # "Incorporate the application manifest with the temporary image and other relevant files into the user-specified application image file.\nThe next step after this one is to start cleaning up."
        n125 = Unbundle By Name(w351) -> ("AppImage Properties.FPGA Properties"=w350:T4, "App Image Info File Path"=w349:path, "Temp Image Path"=w348:path, "AppImage Path"=w347:path)
        n126 = call "rad_PackageImage.vi"("AppImage Properties.FPGA Properties"=w350, "error in (no error)"=w353, "AppImage Path"=w347, "Temp Image Path"=w348, "App Image Info File Path"=w349) -> ("error out"=w352:errorcluster)  [unwired: 6 in]
      }
      frame "Cleanup" {
        # "We finished the image retrieval process, let the user know the final status.\nThe next step after this one is to finish cleaning up."
        n127 = call "Util_Progress Close Progress Popup.vi"("error in (no error)"=w355) -> ("error out"=w356:errorcluster)  [unwired: 10 in]
        n128 = Unbundle By Name(w356) -> ("code"=w359:i32, "source"=w360:string)
        n129 = case shown="0, 221" w359 {
          selector: w359 -> [_ _ w371]
          tunnel: w360 -> [_ _ w374]
          tunnel: ["Application image retrieval successful." ("source") "Error 56 Occurred: Unable to establish communication with the target.  Verify that your network settings are valid." ("source") w373] -> w358
          tunnel: [w363 w366 w369] -> w357
          tunnel: w356 -> [w364 w367 w370]
          frame 0, 221 {
            n130 = call <vilib>:"Clear Errors.vi"("error in (no error)"=w364) -> ("error out"=w363:errorcluster)  [unwired: 5 in, 1 out]
          }
          frame 56 {
            n131 = call <vilib>:"Clear Errors.vi"("error in (no error)"=w367) -> ("error out"=w366:errorcluster)  [unwired: 5 in, 1 out]
          }
          frame Default {
            n132 = Format Into String(format string="Application Image Retrieval Error:\\r\\n %s - %d", w374, w371) -> (resulting string=w373:string)  [unwired: 2 in, 1 out]
            n133 = call <vilib>:"Clear Errors.vi"("error in (no error)"=w370) -> ("error out"=w369:errorcluster)  [unwired: 5 in, 1 out]
          }
        }
        n134 = One Button Dialog(message=w358) -> ()  [unwired: 2 out]
      }
      frame "Exit" {
        # "Remove the temporary folder and all contents (including the temporary image) created in the various stages of this process.\nThis is the final step."
        n135 = Unbundle By Name(w375) -> ("Temp Image Folder"=w377:path)
        n136 = Delete(path (use dialog)=w377, entire hierarchy (F)=TRUE) -> ()  [unwired: 1 in, 5 out]
      }
    }
  }
  "error out" <- w7
  n137 = Unbundle By Name(w6) -> ("AppImage Path"=→"New App Image Path":path)
